vi "Go To Coarse Axis Position (um).vi"(8 "error in (no error)":errorcluster, 10 "Coarse Axis Position (um)":dbl[unit], 11 "GPIB # (in): def. 6":string="6") -> (0 "error out":errorcluster, 3 "GPIB # (out)":string)   [LabVIEW 2015]
uses:
  mc2mc4.llb/MC2/MC4 Wait&ParseSRQ.vi
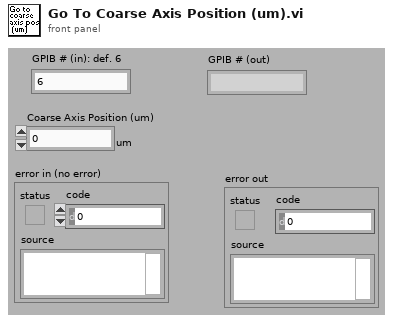
[diagram p1: front panel]
types:
  T1 = enum16{"fine axis move complete", "coarse axis move complete", "either axis move complete", "an axis has reached travel limit"}
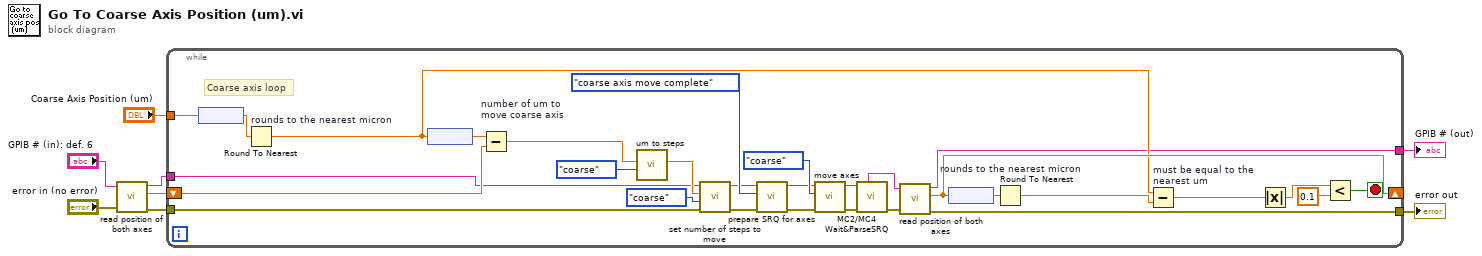
[diagram p0: block diagram]
diagram:
  n1 = call "read position of both axes.vi"("GPIB # (in): def. 6"="GPIB # (in): def. 6", "error in (no error)"="error in (no error)") -> ("GPIB # (out)"=w2:string, "coarse axis (um)"=w4:ext[unit], "error out"=w5:errorcluster)  [unwired: 6 out]
  n2 = while {
    tunnel: "Coarse Axis Position (um)" -> [w25]
    tunnel: w5 -> [w33]
    tunnel: [w32] -> w8
    shift-right: [w21] -> _
    shift-left: w4 -> [w31]
    tunnel: w2 -> [w14]
    tunnel: [w9] -> w1
    stop <- w15 stop-if-true
    # "Coarse axis loop"
    n3 = node(w25) -> (w24:dbl)
    n4 = Round To Nearest "rounds to the nearest micron"(number=w24) -> (nearest integer value=w19:dbl)
    n5 = node(w19) -> (w23:dbl[unit])
    n6 = Subtract "number of um to\nmove coarse axis"(x=w23, y=w31) -> (x-y=w37:ext[unit])
    n7 = call "um to steps.vi"("axis (default = fine)"=enum16{"fine", "coarse"}."coarse", "position (microns)"=w37) -> ("steps"=w36:dbl)  [unwired: 9 out]
    n8 = call "set number of steps to move.vi"("error in"=w33, "axis (def: fine)"=enum16{"fine", "coarse"}."coarse", "number of steps to set"=w36, "GPIB # (in): def. 6"=w14) -> ("error out"=w30:errorcluster, "GPIB # (out)"=w13:string)  [unwired: 6 out]
    n9 = call "prepare SRQ for axes.vi"("error in (no error)"=w30, "category"=T1."coarse axis move complete", "GPIB # (in): def. 6"=w13) -> ("error out"=w29:errorcluster, "GPIB # (out):"=w12:string)  [unwired: 7 out]
    n10 = call "move axes.vi"("error in"=w29, "stage to move"=enum16{"both", "fine", "coarse"}."coarse", "GPIB # (in): def. 6"=w12) -> ("error out"=w28:errorcluster, "GPIB # (out)"=w11:string)  [unwired: 7 out]
    n11 = call "MC2/MC4 Wait&ParseSRQ.vi"("error in (no error)"=w28, "GPIB # (in): def. 6"=w11) -> ("error out"=w27:errorcluster, "GPIB #(out): def. 6"=w10:string)  [unwired: 8 out]
    n12 = call "read position of both axes.vi"("GPIB # (in): def. 6"=w10, "error in (no error)"=w27) -> ("GPIB # (out)"=w9:string, "coarse axis (um)"=w21:ext[unit], "error out"=w32:errorcluster)  [unwired: 6 out]
    n13 = node(w21) -> (w22:ext)
    n14 = Round To Nearest "rounds to the nearest micron"(number=w22) -> (nearest integer value=w20:ext)
    n15 = Subtract "must be equal to the\nnearest um"(x=w19, y=w20) -> (x-y=w16:ext)
    n16 = Absolute Value(x=w16) -> (abs(x)=w18:ext)
    n17 = Less?(x=w18, y=0.1) -> (x < y?=w15:bool)
  }
  "error out" <- w8
  "GPIB # (out)" <- w1
